vi "9_nov_LOOP_2.vi"() -> ()   [LabVIEW 2020]
uses:
  <instrlib>/Agilent B2900 Series/Public/Configure/Measurement/Configure Measurement (Resistance).vi
  <instrlib>/Agilent B2900 Series/Public/Data/Read Measurement Result (Single Point).vi
  <instrlib>/Agilent B2900 Series/Agilent B2900 Series.lvlib
panel:
  out "Voltage":dbl(graph)
  out "Current":dbl(graph)
  out "XY Graph":cluster{"X":dbl[], "Y":dbl[]}[](graph)
  in  "stop":bool
  out "Measured Current (A)":dbl
  out "Measured Voltage (Volts)":dbl
  in  "Enable Current Measurement (T: Enable)":bool=TRUE
  in  "Enable Voltage Measurement (T: Enable)":bool=TRUE
  in  "Enable Resistance Measurement (F: Disable)":bool
  in  "SELECT DEVICE":refnum<visa-resource-name>="COM1"
  out "Measured Resistance (ohms)":dbl
  # "Configuration"
  # "MEASURED VALUES"
  # "ENABLE MODES"
  # "Y"
  # "X"
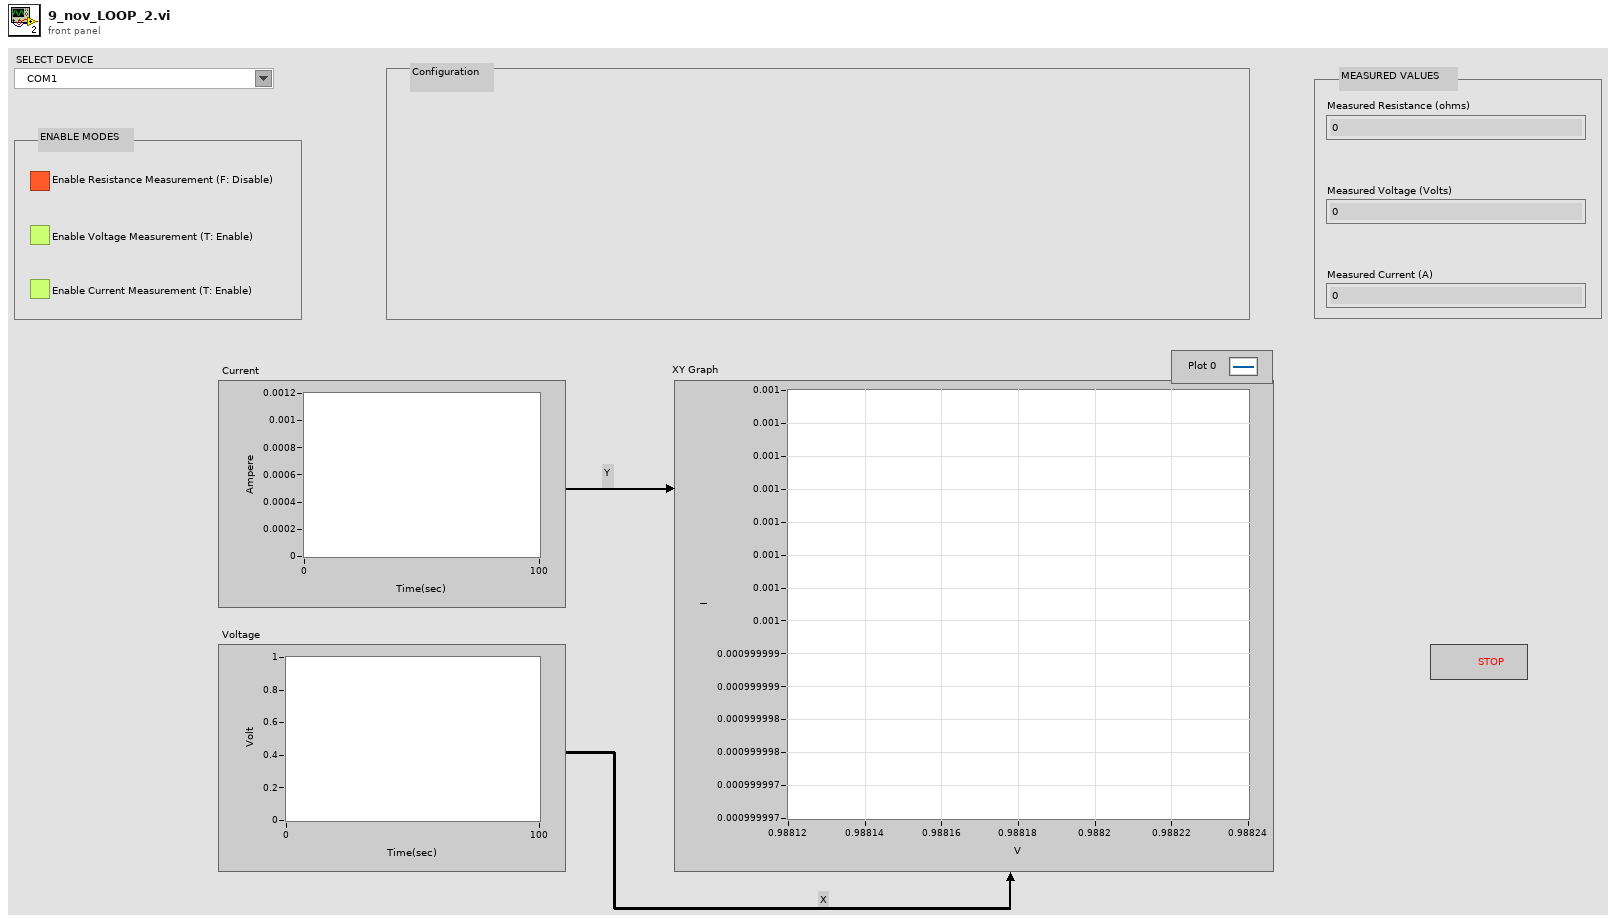
[diagram p1: front panel]
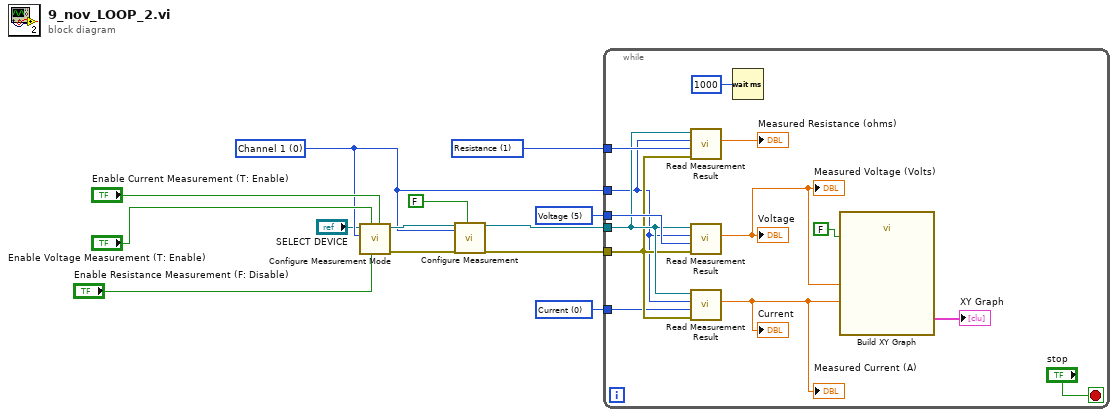
[diagram p0: block diagram]
diagram:
  w3 = 0 items=["Current", "Resistance", "Source Output Setting", "Status", "Time", "Voltage"] ("Data Mode (5: Voltage)")
  w6 = 5 items=["Current", "Resistance", "Source Output Setting", "Status", "Time", "Voltage"] ("Data Mode (5: Voltage)")
  w2 = 0 items=["Channel 1", "Channel 2"] ("Channel (0: Channel 1)")
  w13 = 1 items=["Current", "Resistance", "Source Output Setting", "Status", "Time", "Voltage"] ("Data Mode (5: Voltage)")
  n1 = call <instrlib>:"Configure Measurement Mode.vi"("Enable Current Measurement (T: Enable)"="Enable Current Measurement (T: Enable)", "Enable Resistance Measurement (F: Disable)"="Enable Resistance Measurement (F: Disable)", "Enable Voltage Measurement (T: Enable)"="Enable Voltage Measurement (T: Enable)", "Channel (0: Channel 1)"=w2, "VISA resource name"="SELECT DEVICE") -> ("error out"=w11:errorcluster, "VISA resource name out"=w12:refnum<visa-resource-name>)  [unwired: 5 in]
  n2 = call-poly <instrlib>:"Configure Measurement.vi"("VISA resource name"=w12, "Channel (0: Channel 1)"=w2, "error in (no error)"=w11, "Enable Resistance Compensation (F: Disable)"=FALSE) -> ("VISA resource name out"=w5:refnum<visa-resource-name>, "error out"=w4:errorcluster)  [unwired: 14 in]
  n3 = while {
    tunnel: w13 -> [w26]
    tunnel: w6 -> [w25]
    tunnel: w5 -> [w24]
    tunnel: w4 -> [w23]
    tunnel: w3 -> [w22]
    tunnel: w2 -> [w21]
    stop <- "stop" stop-if-true
    n4 = call-poly <instrlib>:"Read Measurement Result.vi"("error in (no error)"=w23, "Data Mode (5: Voltage)"=w26, "Channel (0: Channel 1)"=w21, "VISA resource name"=w24) -> ("Measurement Result"=→"Measured Resistance (ohms)":dbl)  [unwired: 5 in, 2 out]
    n5 = call-poly <instrlib>:"Read Measurement Result.vi"("error in (no error)"=w23, "Data Mode (5: Voltage)"=w25, "Channel (0: Channel 1)"=w21, "VISA resource name"=w24) -> ("Measurement Result"=w14:dbl)  [unwired: 5 in, 2 out]
    "Measured Voltage (Volts)" <- w14
    "Voltage" <- w14
    n6 = call-poly <instrlib>:"Read Measurement Result.vi"("error in (no error)"=w23, "Data Mode (5: Voltage)"=w22, "Channel (0: Channel 1)"=w21, "VISA resource name"=w24) -> ("Measurement Result"=w15:dbl)  [unwired: 5 in, 2 out]
    "Measured Current (A)" <- w15
    "Current" <- w15
    n7 = Wait (ms)(milliseconds to wait=u32 1000) -> ()  [unwired: 1 out]
    n8 = call "Build XY Graph"("Reset"=FALSE, "Y Input"=w15, "X Input"=w14) -> ("XY Graph"=→"XY Graph":cluster{"X":dbl[], "Y":dbl[]}[])  [unwired: 7 in, 1 out]
  }
